vi "Get Maximum Number Ring Exposure Times.vi"(11 "number":i32) -> (2 "function return":u32, 3 "number out":i32)   [LabVIEW 2018, in "AndorSDK.lvlib"]
doc: "EXPNETTYPE unsigned int WINAPI GetMaximumNumberRingExposureTimes(int * number);"
uses:
  AndorSDK.lvlib
  ATMCD32D.dll
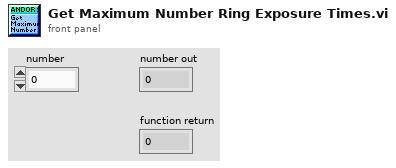
[diagram p1: front panel]
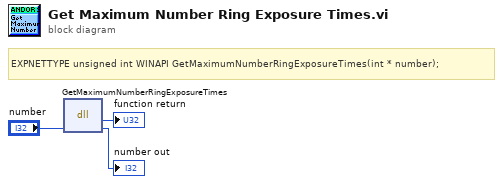
[diagram p0: block diagram]
diagram:
  # "EXPNETTYPE unsigned int WINAPI GetMaximumNumberRingExposureTimes(int * number);"
  n1 = dll-call lib="PTH2babs E\nPersönliches02 - Arbeit03-HiwijobsLabviewCodelibANDOR\tAndor SDK\nATMCD32D.*" fn="GetMaximumNumberRingExposureTimes"("number"="number") -> (→"function return":u32, "number"=→"number out":i32)  [unwired: 3 in, 2 out]
